vi "Test HVPS.vi"() -> ()   [LabVIEW 2013, in "SR 3XX HVPS.lvclass"]
uses:
  SR 3XX HVPS/SR 3XX HVPS.lvclass
  SR 3XX HVPS/SR 3XX HVPS.lvclass/SR 3XX HVPS.ctl
  SR 3XX HVPS/Write GPIB Addr.vi
panel:
  in  "VLIM In":sgl
  out "ITRP":sgl
  out "ILIM":sgl
  out "VLIM":sgl
  in  "stop":bool
  out "VOUT":sgl
  out "SerialPollStat":T1
  out "StdEvntStatus":T2
  out "VSET Out":sgl
  in  "VSET In":sgl
  in  "pow":bool
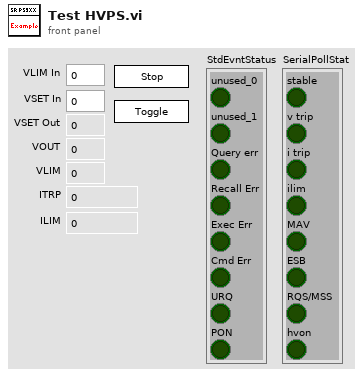
[diagram p1: front panel]
types:
  T1 = cluster{"stable":bool, "v trip":bool, "i trip":bool, "ilim":bool, "MAV":bool, "ESB":bool, "RQS/MSS":bool, "hvon":bool}
  T2 = cluster{"unused_0":bool, "unused_1":bool, "Query err":bool, "Recall Err":bool, "Exec Err":bool, "Cmd Err":bool, "URQ":bool, "PON":bool}
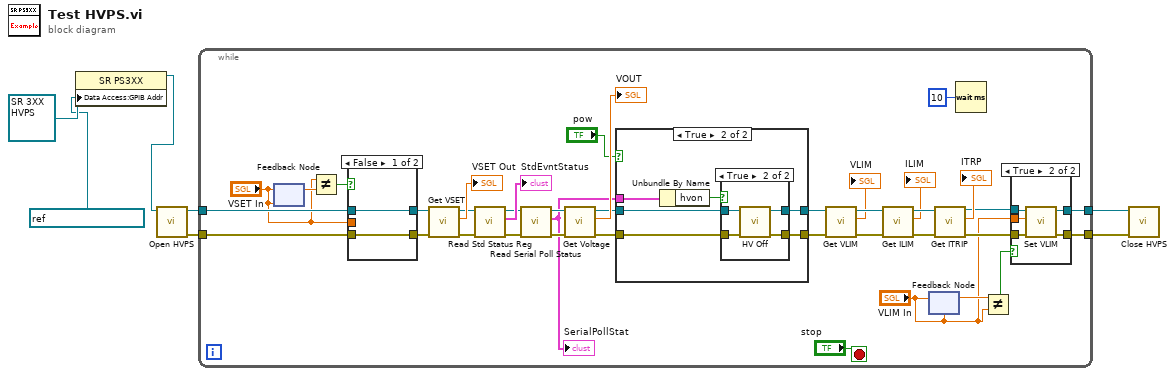
[diagram p0: block diagram]
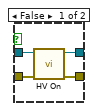
[diagram p4: hidden frame]
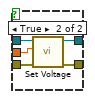
[diagram p5: hidden frame]
diagram:
  n1 = property class="SR PS3XX"(reference=refnum<class "SR 3XX HVPS.lvclass"> refnum ("SR 3XX HVPS in"), "Data Access:GPIB Addr"=refnum<visa-resource-name> "GPIB0::11::INSTR" ("GPIB Resc")) -> (reference out=w2:refnum<class "SR 3XX HVPS.lvclass">)  [unwired: 1 in, 1 out]
  n2 = call-dynamic "Open HVPS.vi"("SR 3XX HVPS in"=w2) -> ("error out"=w6:errorcluster, "SR 3XX HVPS out"=w7:refnum<class "SR 3XX HVPS.lvclass">)  [unwired: 9 in]
  n3 = while {
    tunnel: w7 -> [w45]
    tunnel: w6 -> [w41]
    tunnel: [w11] -> w5
    tunnel: [w10] -> w4
    stop <- "stop" stop-if-true
    n4 = feedback-in #1("VSET In") -> ()
    n5 = feedback #1("VSET In") -> (w44:sgl)
    n6 = Not Equal?(x="VSET In", y=w44) -> (x != y?=w42:bool)
    n7 = case shown="False" w42 {
      tunnel: "VSET In" -> [_ w75]
      tunnel: w45 -> [w70 w74]
      tunnel: w41 -> [w69 w73]
      tunnel: [w70 w72] -> w40
      tunnel: [w69 w71] -> w39
      frame False {
      }
      frame True {
        n8 = call-dynamic "Set Voltage.vi"("error in"=w73, "Voltage"=w75, "SR 3XX HVPS in"=w74) -> ("error out"=w71:errorcluster, "SR 3XX HVPS out"=w72:refnum<class "SR 3XX HVPS.lvclass">)  [unwired: 7 in]
      }
    }
    n9 = call "Get VSET.vi"("error in"=w39, "SR 3XX HVPS in"=w40) -> ("error out"=w36:errorcluster, "VSET"=→"VSET Out":sgl, "SR 3XX HVPS out"=w37:refnum<class "SR 3XX HVPS.lvclass">)  [unwired: 7 in]
    n10 = call "Read Std Status Reg.vi"("error in"=w36, "SR 3XX HVPS in"=w37) -> ("error out"=w33:errorcluster, "StdEvntStatus"=→"StdEvntStatus":T2, "SR 3XX HVPS out"=w34:refnum<class "SR 3XX HVPS.lvclass">)  [unwired: 7 in]
    n11 = call "Read Serial Poll Status.vi"("error in"=w33, "SR 3XX HVPS in"=w34) -> ("error out"=w31:errorcluster, "SerialPollStat"=w26:T1, "SR 3XX HVPS out"=w32:refnum<class "SR 3XX HVPS.lvclass">)  [unwired: 7 in]
    "SerialPollStat" <- w26
    n12 = call-dynamic "Get Voltage.vi"("error in"=w31, "SR 3XX HVPS in"=w32) -> ("error out"=w27:errorcluster, "VOUT"=→"VOUT":sgl, "SR 3XX HVPS out"=w29:refnum<class "SR 3XX HVPS.lvclass">)  [unwired: 7 in]
    n13 = case shown="True" "pow" {
      tunnel: w29 -> [w54 w58]
      tunnel: w27 -> [w53 w57]
      tunnel: w26 -> [_ w60]
      tunnel: [w54 w56] -> w24
      tunnel: [w53 w55] -> w21
      frame False {
      }
      frame True {
        n14 = Unbundle By Name(w60) -> ("hvon"=w59:bool)
        n15 = case shown="True" w59 {
          tunnel: w58 -> [w64 w68]
          tunnel: w57 -> [w63 w67]
          tunnel: [w62 w66] -> w56
          tunnel: [w61 w65] -> w55
          frame False {
            n16 = call "HV On.vi"("error in"=w63, "SR 3XX HVPS in"=w64) -> ("error out"=w61:errorcluster, "SR 3XX HVPS out"=w62:refnum<class "SR 3XX HVPS.lvclass">)  [unwired: 8 in]
          }
          frame True {
            n17 = call "HV Off.vi"("error in"=w67, "SR 3XX HVPS in"=w68) -> ("error out"=w65:errorcluster, "SR 3XX HVPS out"=w66:refnum<class "SR 3XX HVPS.lvclass">)  [unwired: 8 in]
          }
        }
      }
    }
    n18 = call "Get VLIM.vi"("error in"=w21, "SR 3XX HVPS in"=w24) -> ("error out"=w20:errorcluster, "VLIM"=→"VLIM":sgl, "SR 3XX HVPS out"=w23:refnum<class "SR 3XX HVPS.lvclass">)  [unwired: 7 in]
    n19 = call "Get ILIM.vi"("error in"=w20, "SR 3XX HVPS in"=w23) -> ("error out"=w19:errorcluster, "ILIM"=→"ILIM":sgl, "SR 3XX HVPS out"=w22:refnum<class "SR 3XX HVPS.lvclass">)  [unwired: 7 in]
    n20 = feedback-in #2("VLIM In") -> ()
    n21 = feedback #2("VLIM In") -> (w14:sgl)
    n22 = call "Get ITRIP.vi"("error in"=w19, "SR 3XX HVPS in"=w22) -> ("error out"=w12:errorcluster, "ITRP"=→"ITRP":sgl, "SR 3XX HVPS out"=w13:refnum<class "SR 3XX HVPS.lvclass">)  [unwired: 7 in]
    n23 = Wait (ms)(milliseconds to wait=u32 10) -> ()  [unwired: 1 out]
    n24 = Not Equal?(x=w14, y="VLIM In") -> (x != y?=w15:bool)
    n25 = case shown="True" w15 {
      tunnel: "VLIM In" -> [_ w52]
      tunnel: w13 -> [w47 w51]
      tunnel: w12 -> [w46 w50]
      tunnel: [w47 w49] -> w11
      tunnel: [w46 w48] -> w10
      frame False {
      }
      frame True {
        n26 = call "Set VLIM.vi"("error in"=w50, "VLIM"=w52, "SR 3XX HVPS in"=w51) -> ("error out"=w48:errorcluster, "SR 3XX HVPS out"=w49:refnum<class "SR 3XX HVPS.lvclass">)  [unwired: 7 in]
      }
    }
  }
  n27 = call-dynamic "Close HVPS.vi"("error in"=w4, "SR 3XX HVPS in"=w5) -> ()  [unwired: 8 in, 2 out]
